vi "XIPIN_S_PDIF_2_0.vi"   [LabVIEW 2017]
doc: "S/PDIF is an audio controller which has interface to master through AXI streaming and to AXI4-Lite.This core works as a transmitter or as a receiver based on the selected mode.\n------------------------------------\n<b>Need License</b> : Yes\n<b>Interface</b> : AXI4 AXI4-Stream"
uses:
  <vilib>/rvi/XilinxIP/XIPIN_XNode/niFpgaXIPIN.xnode
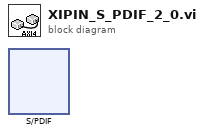
[diagram p0: block diagram]
diagram:
  n1 = xnode ("S/PDIF")() -> ()
